vi "Test Func Generator API.vi"() -> ()   [LabVIEW 2016]
doc: "Func Generator API Tester."
uses:
  <vilib>/Utility/miscctls.llb/LVPointTypeDef.ctl
  <vilib>/Utility/error.llb/DialogType.ctl
  Instrument Setting.ctl
  Func Generator.lvlib
panel:
  in  "Serial Configuration":T1={"Baud Rate"=9600, "Parity"=0, "Data Bits"=8, "Flow Control"=4} {"Flow Control" items=["None", "XON/XOFF", "RTS/CTS", "XON/XOFF & RTS/CTS", "DTR/DSR", "XON/XOFF & DTR/DSR"]; "Data Bits" items=["7"=7, "8"=8]; "Parity" items=["None", "Odd", "Even", "Mark", "Space"]; "Baud Rate" items=["300"=300, "600"=600, "1200"=1200, "2400"=2400, "4800"=4800, "9600"=9600, "19200"=19200]}
  in  "REQ Close Ref":bool
  in  "REQ Self Test":bool
  in  "Freq Sweep Setting":T2={"Sweep Spacing (0: Linear)"=0, "Sweep Time (1.00 s)"=1.0, "Stop  Frequency (1000.0 Hz)"=1000.0, "Start Frequency (100.0 Hz)"=100.0, "Enable/Disable Freq Sweep"=FALSE} {"Start Frequency (100.0 Hz)" format="%#.6g"; "Stop  Frequency (1000.0 Hz)" format="%#.6g"; "Sweep Time (1.00 s)" format="%#.6g"; "Sweep Spacing (0: Linear)" items=["Linear", "Logarithmic"]}
  in  "REQ Config Freq Sweep":bool
  in  "Std Waveform Setting":T3={"Waveform Function (1: Sine)"=1, "Frequency (1000 Hz)"=1000.0, "Amplitude (1)"=1.0, "Unit (0: Vpp)"=0, "DC Offset (0.00 V)"=0.0} {"Unit (0: Vpp)" items=["Vpp", "Vrms", "dB"]; "Waveform Function (1: Sine)" items=["DC", "Sine", "Square", "Triangle", "Ramp", "Pulse", "Noise", "Sinc", "Negative Ramp", "Exponential Rise", "Exponential Fall", "Cardiac"]}
  in  "REQ Config Std Waveform":bool
  in  "Impedance (0: 50 Ohms)":u16(ring) items=["50 Ohms", "High Impedance", "User Defined"]
  in  "User-Defined Impedance (50 Ohms)":dbl=50.0 min=1.0 max=10000.0 format="%.2f"
  in  "REQ Set Output Impedance":bool
  in  "Output":bool
  in  "REQ Enable Output":bool
  in  "DAQ Type":enum16{"Hardware", "Simulation"}(ring)
  out "Connect?":bool
  in  "Instrument Address":refnum<visa-resource-name>
  in  "REQ Initialize Hardware":bool
  in  "Show Diagram on Init":bool
  in  "Show Block Diagram":bool
  in  "Stop Module":bool
  in  "Start Module":bool
  in  "Hide Module Panel":bool
  in  "Show Module Panel":bool
  out "Status":string
  out "Module Running?":bool
  # "This VI tests the API for the Module."
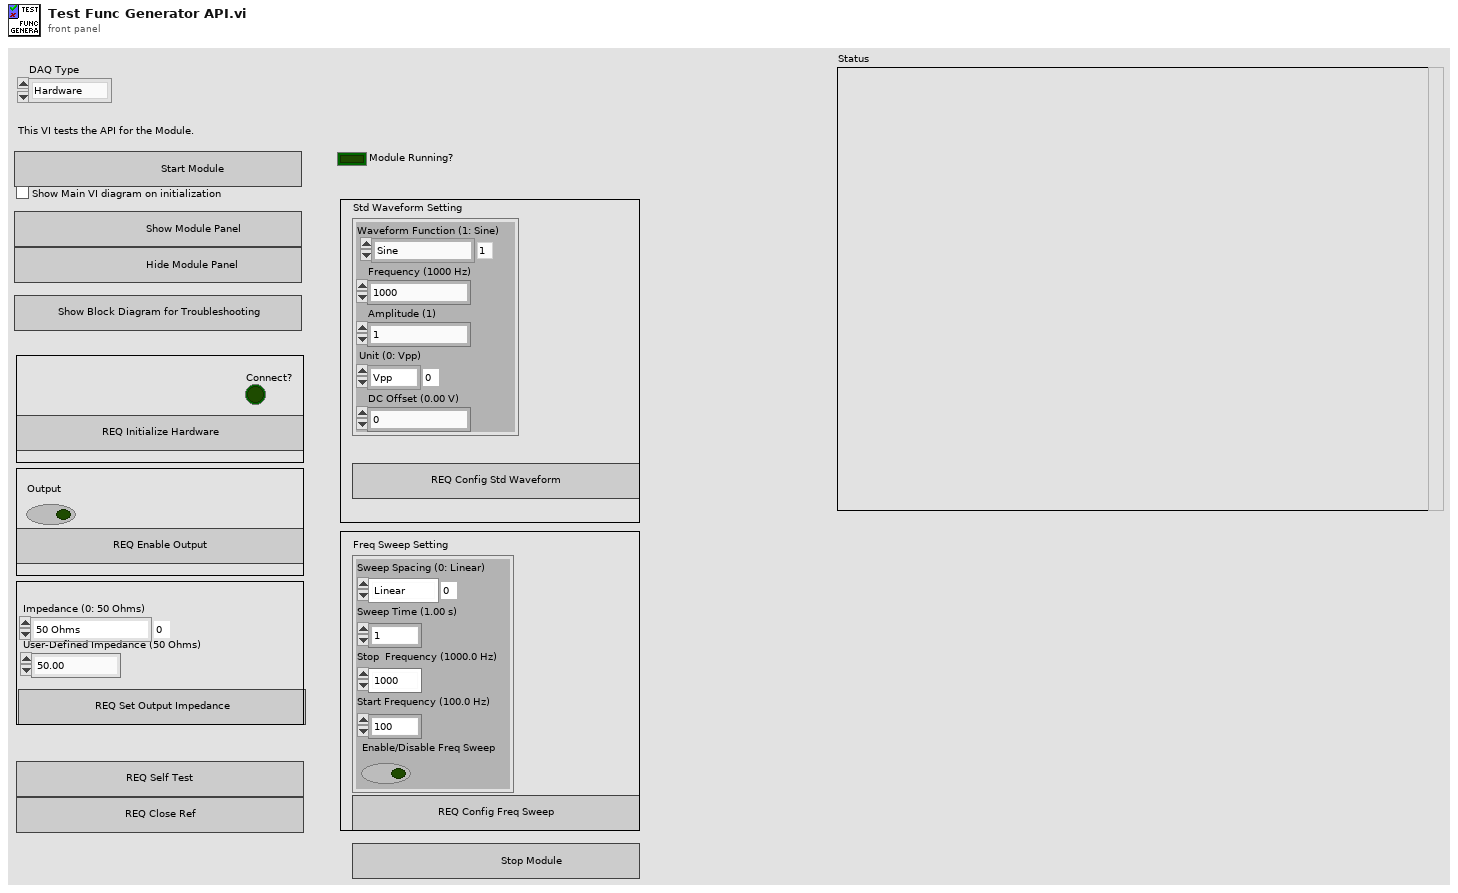
[diagram p1: front panel]
types:
  T1 = cluster{"Baud Rate":u32, "Parity":u16, "Data Bits":u16, "Flow Control":u16}
  T2 = cluster{"Sweep Spacing (0: Linear)":u16, "Sweep Time (1.00 s)":dbl, "Stop  Frequency (1000.0 Hz)":dbl, "Start Frequency (100.0 Hz)":dbl, "Enable/Disable Freq Sweep":bool}
  T3 = cluster{"Waveform Function (1: Sine)":u16, "Frequency (1000 Hz)":dbl, "Amplitude (1)":dbl, "Unit (0: Vpp)":u16, "DC Offset (0.00 V)":dbl}
  T4 = typedef "LVPointTypeDef.ctl" = cluster{"Horizontal":i16, "Vertical":i16}
  T5 = typedef "Func Generator.lvlib/Broadcast Events--cluster.ctl" = cluster{"Module Did Init":refnum<user-event>, "Status Updated":refnum<user-event>, "Error Reported":refnum<user-event>, "Module Did Stop":refnum<user-event>, "Update Module Execution Status":refnum<user-event>}
  T6 = typedef "Func Generator.lvlib/Instrument Setting.ctl" = cluster{"Ref":variant, "Serial":cluster{"Baud Rate":u32, "Parity":u16, "Data Bits":u16, "Flow Control":u16}}
  T7 = typedef "DialogType.ctl" = u16
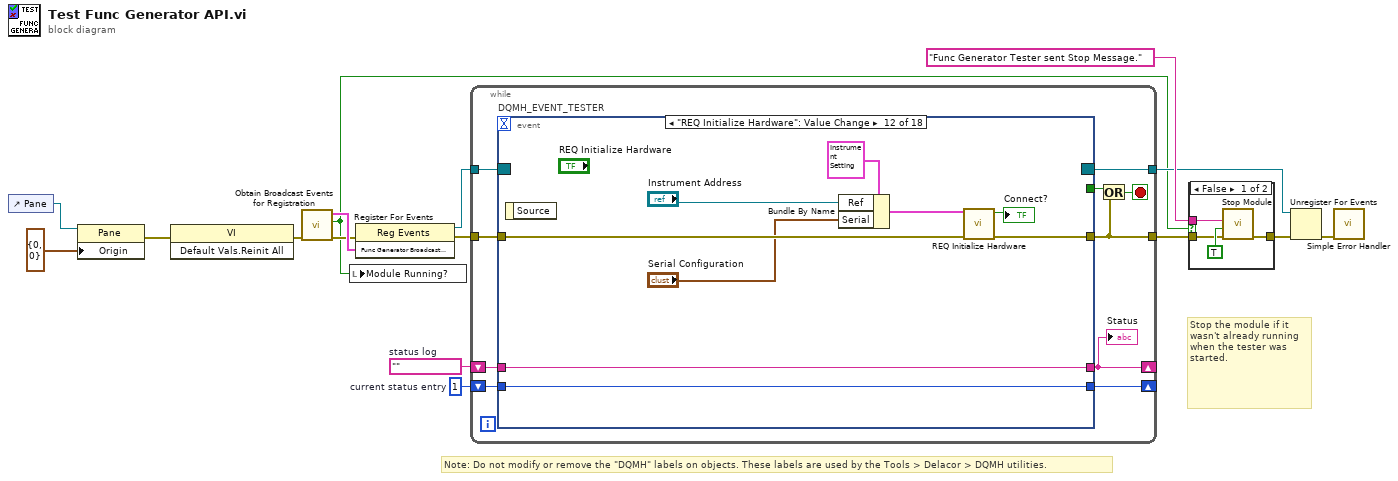
[diagram p0: block diagram]
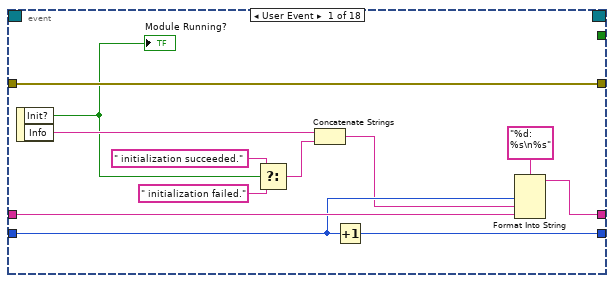
[diagram p3: hidden frame]
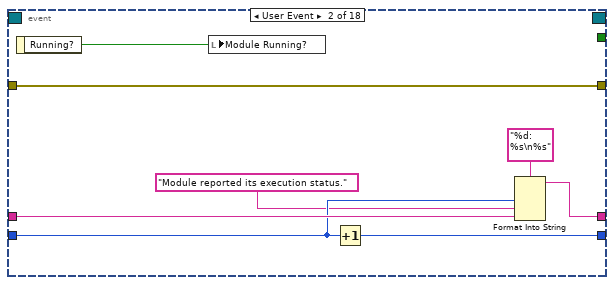
[diagram p4: hidden frame]
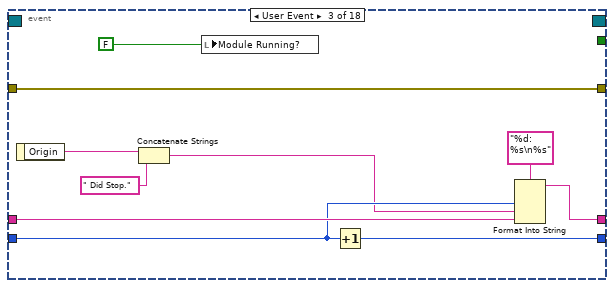
[diagram p5: hidden frame]
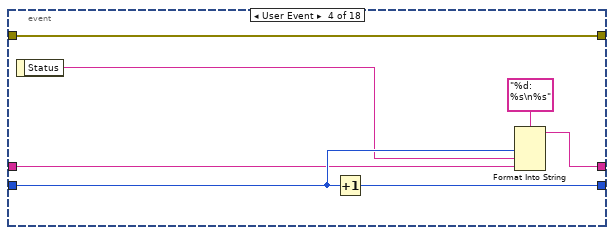
[diagram p6: hidden frame]
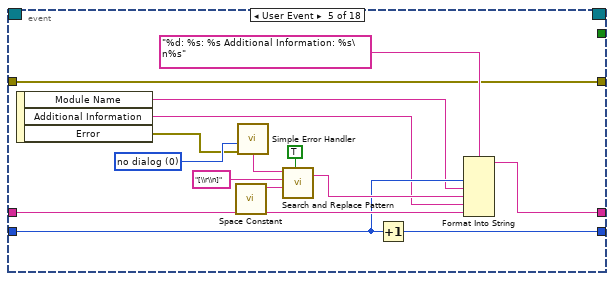
[diagram p7: hidden frame]
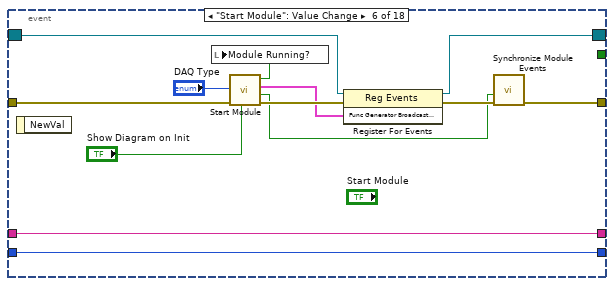
[diagram p8: hidden frame]
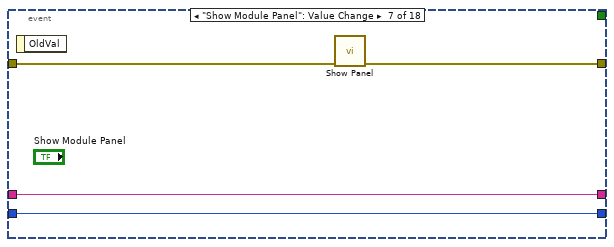
[diagram p9: hidden frame]
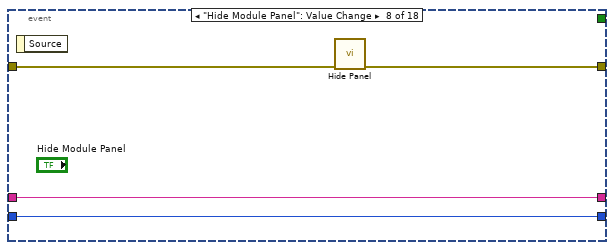
[diagram p10: hidden frame]
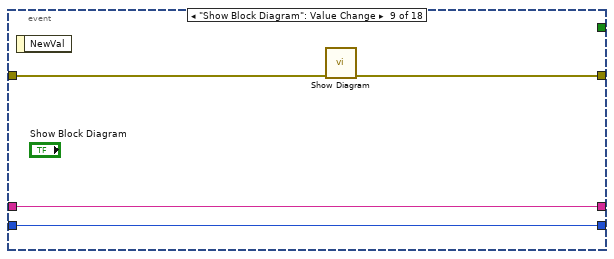
[diagram p11: hidden frame]
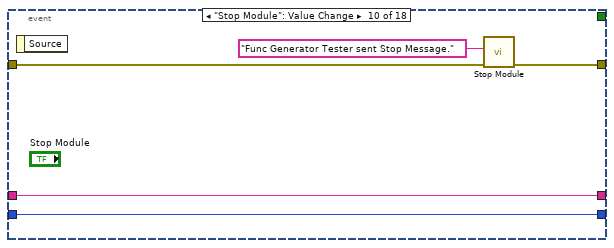
[diagram p12: hidden frame]
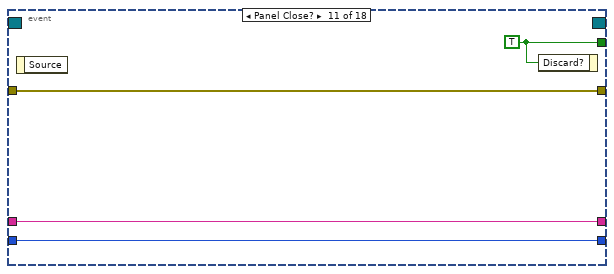
[diagram p13: hidden frame]
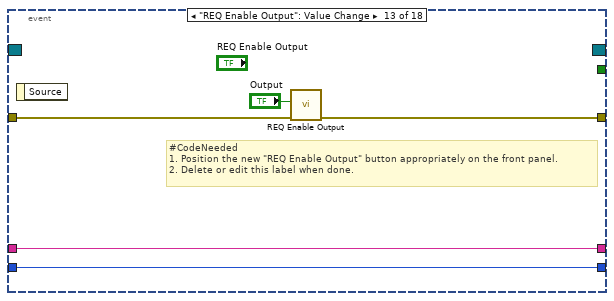
[diagram p14: hidden frame]
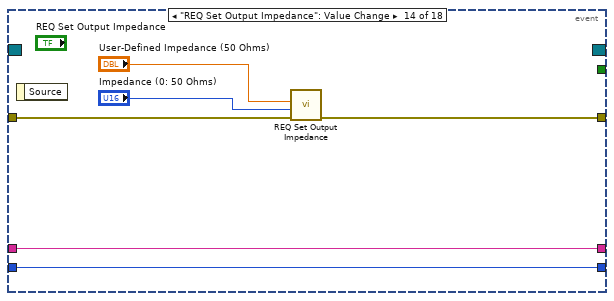
[diagram p15: hidden frame]
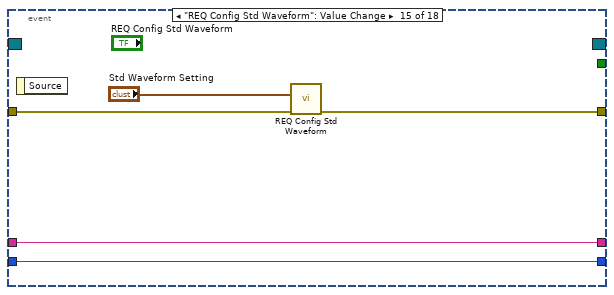
[diagram p16: hidden frame]
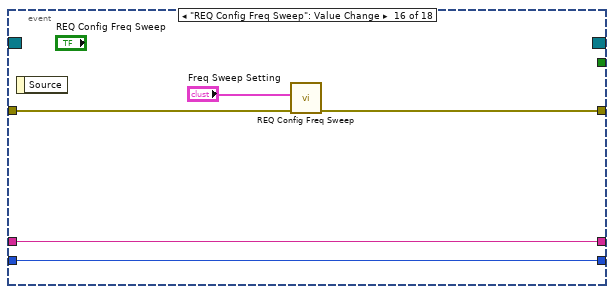
[diagram p17: hidden frame]
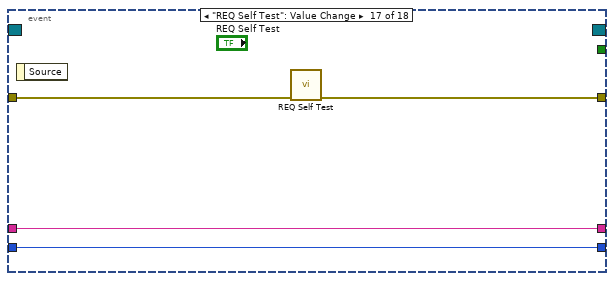
[diagram p18: hidden frame]
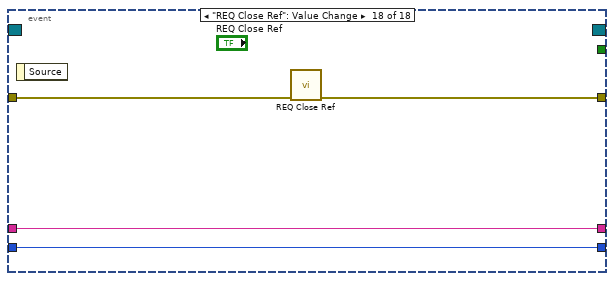
[diagram p19: hidden frame]
diagram:
  w13 = 1  # current status entry
  w14 = ""  # status log
  # "Stop the module if it wasn't already running when the tester was started."
  # "Note: Do not modify or remove the \"DQMH\" labels on objects. These labels are used by the Tools > Delacor > DQMH utilities."
  n1 = control-ref of="Pane"() -> (w2:refnum<vi>)
  n2 = property class="Pane"(reference=w2, "Origin"=T4 {"Horizontal"=0, "Vertical"=0}) -> (error out=w3:errorcluster)  [unwired: 1 in, 1 out]
  n3 = invoke class="VI" method="Default Vals.Reinit All"(error in=w3) -> (error out=w8:errorcluster)  [unwired: 2 in, 2 out]
  n4 = call "Obtain Broadcast Events for Registration.vi"("error in"=w8) -> ("error out"=w7:errorcluster, "Already running?"=w6:bool, "Func Generator Broadcast Events"=w11:T5)  [unwired: 8 in]
  n5 = local write "Module Running?"(w6) -> ()
  n6 = register-events(error in=w7, w11) -> (reference out=w10:refnum<event-registration>, error out=w12:errorcluster)  [unwired: 1 in]
  n7 = while {
    tunnel: w10 -> [w26]
    tunnel: [w17] -> w5
    shift-right: [w21] -> _
    shift-left: w14 -> [w23]
    shift-right: [w22] -> _
    shift-left: w13 -> [w24]
    tunnel: w12 -> [w19]
    tunnel: [w18] -> w9
    stop <- w20 stop-if-true
    n8 = event "DQMH_EVENT_TESTER" shown="[11] \"REQ Initialize Hardware\": Value Change" {
      selector: w26 -> [_ _ _ _ _ w85 _ _ _ _ _ _ _ _ _ _ _ _]
      dyn-events: [_ _ _ _ _ w84 _ _ _ _ _ _ _ _ _ _ _ _] -> w18
      timeout: _ -> [_ _ _ _ _ _ _ _ _ _ _ _ _ _ _ _ _ _]
      tunnel: [_ _ _ _ _ _ _ _ _ _ w112 _ _ _ _ _ _ _] -> w25
      tunnel: [w38 w40 w47 w57 w67 w83 w95 w99 w100 w106 w109 w118 w123 w129 w134 w139 w143 w147] -> w17
      tunnel: w24 -> [w35 w44 w54 w60 w70 w88 w93 w97 w101 w107 w110 w119 w124 w130 w135 w140 w144 w148]
      tunnel: w23 -> [w36 w45 w55 w59 w71 w89 w94 w98 w102 w108 w111 w120 w125 w131 w136 w141 w145 w149]
      tunnel: [w33 w42 w52 w61 w69 w89 w94 w98 w102 w108 w111 w120 w125 w131 w136 w141 w145 w149] -> w21
      tunnel: [w34 w43 w53 w63 w68 w88 w93 w97 w101 w107 w110 w119 w124 w130 w135 w140 w144 w148] -> w22
      tunnel: w19 -> [w38 w40 w47 w57 w67 w82 w92 w96 w103 w104 w109 w121 w126 w132 w137 w142 w146 w150]
      event User Event {
        n9 = event-data() -> ("Init?"=w30:bool, "Info"=w32:string)  [unwired: 1 in]
        "Module Running?" <- w30
        n10 = Select(t=" initialization succeeded.", s=w30, f=" initialization failed.") -> (s? t:f=w27:string)
        n11 = Concatenate Strings(w32, w27) -> (w31:string)
        n12 = Increment(x=w35) -> (x+1=w34:i32)
        n13 = Format Into String(format string="%d: %s\n%s", w35, w31, w36) -> (resulting string=w33:string)  [unwired: 2 in, 1 out]
      }
      event User Event {
        n14 = event-data() -> ("Running?"=w39:bool)  [unwired: 1 in]
        n15 = local write "Module Running?"(w39) -> ()
        n16 = Increment(x=w44) -> (x+1=w43:i32)
        n17 = Format Into String(format string="%d: %s\n%s", w44, "Module reported its execution status.", w45) -> (resulting string=w42:string)  [unwired: 2 in, 1 out]
      }
      event User Event {
        n18 = event-data() -> ("Origin"=w51:string)  [unwired: 1 in]
        n19 = Concatenate Strings(w51, " Did Stop.") -> (w50:string)
        n20 = local write "Module Running?"(FALSE ("Module Did Init?")) -> ()
        n21 = Increment(x=w54) -> (x+1=w53:i32)
        n22 = Format Into String(format string="%d: %s\n%s", w54, w50, w55) -> (resulting string=w52:string)  [unwired: 2 in, 1 out]
      }
      event User Event {
        n23 = event-data() -> ("Status"=w58:string)  [unwired: 1 in]
        n24 = Increment(x=w60) -> (x+1=w63:i32)
        n25 = Format Into String(format string="%d: %s\n%s", w60, w58, w59) -> (resulting string=w61:string)  [unwired: 2 in, 1 out]
      }
      event User Event {
        w72 = T7 0 items=["no dialog", "OK message", "continue or stop message", "OK message + warnings", "continue/stop + warnings"] ("type of dialog (OK msg:1)")
        n26 = event-data() -> ("Module Name"=w66:string, "Additional Information"=w65:string, "Error"=w64:errorcluster)  [unwired: 1 in]
        n27 = call <vilib>:"Space Constant.vi"() -> ("String"=w76:string)
        n28 = call <vilib>:"Simple Error Handler.vi"("type of dialog (OK msg:1)"=w72, "error in (no error)"=w64) -> ("message"=w73:string)  [unwired: 3 in, 4 out]
        n29 = call <vilib>:"Search and Replace Pattern.vi"("string"=w73, "regular expression (\"\")"="[\\r\\n]" ("regular expression (\"\")"), "replace string (\"\")"=w76, "replace all? (F)"=TRUE ("replace all CR/LF with spaces")) -> ("result string"=w74:string)  [unwired: 1 in, 1 out]
        n30 = Increment(x=w70) -> (x+1=w68:i32)
        n31 = Format Into String(format string="%d: %s: %s Additional Information: %s\n%s", w70, w66, w74, w65, w71) -> (resulting string=w69:string)  [unwired: 2 in, 1 out]
      }
      event "Start Module": Value Change {
        n32 = event-data() -> ()  [unwired: 1 in, 1 out]
        n33 = call "Start Module.vi"("Show Main VI Diagram on Init (F)"="Show Diagram on Init", "error in"=w82, "DAQ Type"="DAQ Type") -> ("error out"=w90:errorcluster, "Wait for Event Sync?"=w87:bool, "Func Generator Broadcast Events"=w86:T5, "Module Was Already Running?"=w81:bool)  [unwired: 5 in]
        n34 = local write "Module Running?"(w81) -> ()
        n35 = register-events(reference=w85, error in=w90, w86) -> (reference out=w84:refnum<event-registration>, error out=w91:errorcluster)
        n36 = call "Synchronize Module Events.vi"("error in"=w91, "Wait for Event Sync?"=w87) -> ("error out"=w83:errorcluster)  [unwired: 9 in]
      }
      event "Show Module Panel": Value Change {
        n37 = event-data() -> ()  [unwired: 1 in, 1 out]
        n38 = call "Show Panel.vi"("error in (no error)"=w92) -> ("error out"=w95:errorcluster)  [unwired: 10 in]
      }
      event "Hide Module Panel": Value Change {
        n39 = event-data() -> ()  [unwired: 1 in, 1 out]
        n40 = call "Hide Panel.vi"("error in (no error)"=w96) -> ("error out"=w99:errorcluster)  [unwired: 10 in]
      }
      event "Show Block Diagram": Value Change {
        n41 = event-data() -> ()  [unwired: 1 in, 1 out]
        n42 = call "Show Diagram.vi"("error in (no error)"=w103) -> ("error out"=w100:errorcluster)  [unwired: 10 in]
      }
      event "Stop Module": Value Change {
        n43 = event-data() -> ()  [unwired: 1 in, 1 out]
        n44 = call "Stop Module.vi"("error in"=w104, "Origin"="Func Generator Tester sent Stop Message.") -> ("error out"=w106:errorcluster)  [unwired: 9 in]
      }
      event Panel Close? {
        w112 = TRUE ("Discard?")
        n45 = event-data() -> ()  [unwired: 1 in, 1 out]
        n46 = event-data("Discard?"=w112) -> ()  [unwired: 1 in, 1 out]
      }
      event "REQ Initialize Hardware": Value Change {
        n47 = event-data() -> ()  [unwired: 1 in, 1 out]
        n48 = Bundle By Name(cluster=T6 {"Ref"=variant, "Serial"={"Baud Rate"=9600, "Parity"=0, "Data Bits"=8, "Flow Control"=4}} ("Connection Setting"), "Ref"="Instrument Address", "Serial"="Serial Configuration") -> (w113:T6)
        n49 = call "REQ Initialize Hardware.vi"("error in"=w121, "Connection Setting"=w113) -> ("error out"=w118:errorcluster, "Connect?"=→"Connect?":bool)  [unwired: 7 in, 1 out]
      }
      event "REQ Enable Output": Value Change {
        # "#CodeNeeded\n1. Position the new \"REQ Enable Output\" button appropriately on the front panel.\n2. Delete or edit this label when done."
        n50 = event-data() -> ()  [unwired: 1 in, 1 out]
        n51 = call "REQ Enable Output.vi"("error in"=w126, "Output"="Output") -> ("error out"=w123:errorcluster)  [unwired: 9 in]
      }
      event "REQ Set Output Impedance": Value Change {
        n52 = event-data() -> ()  [unwired: 1 in, 1 out]
        n53 = call "REQ Set Output Impedance.vi"("error in"=w132, "Impedance (0: 50 Ohms)"="Impedance (0: 50 Ohms)", "User-Defined Impedance (50 Ohms)"="User-Defined Impedance (50 Ohms)") -> ("error out"=w129:errorcluster)  [unwired: 8 in]
      }
      event "REQ Config Std Waveform": Value Change {
        n54 = event-data() -> ()  [unwired: 1 in, 1 out]
        n55 = call "REQ Config Std Waveform.vi"("error in"=w137, "Std Waveform Setting"="Std Waveform Setting") -> ("error out"=w134:errorcluster)  [unwired: 9 in]
      }
      event "REQ Config Freq Sweep": Value Change {
        n56 = event-data() -> ()  [unwired: 1 in, 1 out]
        n57 = call "REQ Config Freq Sweep.vi"("error in"=w142, "Freq Sweep Setting"="Freq Sweep Setting") -> ("error out"=w139:errorcluster)  [unwired: 9 in]
      }
      event "REQ Self Test": Value Change {
        n58 = event-data() -> ()  [unwired: 1 in, 1 out]
        n59 = call "REQ Self Test.vi"("error in"=w146) -> ("error out"=w143:errorcluster)  [unwired: 10 in]
      }
      event "REQ Close Ref": Value Change {
        n60 = event-data() -> ()  [unwired: 1 in, 1 out]
        n61 = call "REQ Close Ref.vi"("error in"=w150) -> ("error out"=w147:errorcluster)  [unwired: 10 in]
      }
    }
    "Status" <- w21
    n62 = Or(x=w25, y=w17) -> (x .or. y?=w20:bool)
  }
  n63 = case shown="False" w6 {
    tunnel: [w154 w155] -> w16
    tunnel: "Func Generator Tester sent Stop Message." ("Origin") -> [w153 _]
    tunnel: w5 -> [w151 w155]
    frame False {
      n64 = call "Stop Module.vi"("error in"=w151, "Wait for Module to Stop? (F)"=TRUE ("Wait for Module to stop?"), "Origin"=w153) -> ("error out"=w154:errorcluster)  [unwired: 8 in]
    }
    frame True {
    }
  }
  n65 = Unregister For Events(event registration refnum=w9, error in=w16) -> (error out=w4:errorcluster)
  n66 = call <vilib>:"Simple Error Handler.vi"("error in (no error)"=w4) -> ()  [unwired: 4 in, 5 out]
